vi "Modbus Property Names.vi"() -> ()   [LabVIEW 2013, in "Modbus Shared.lvlib"]
uses:
  Shared/Modbus Shared.lvlib
panel:
  in  "Modbus Items FIFO Indexes":string="Modbus Items FIFO Indexes"
  in  "Modbus Items Channels References":string="Modbus Items Channels References"
  in  "Modbus Items":string="Modbus Items"
  in  "Modbus General Settings":string="Modbus General Settings"
  in  "Modbus Configuration File Content":string="Modbus Configuration File Content"
  in  "Modbus Configuration File Path":string="Modbus Configuration File Path"
  in  "Modbus Configuration File MD5":string="Modbus Configuration File MD5"
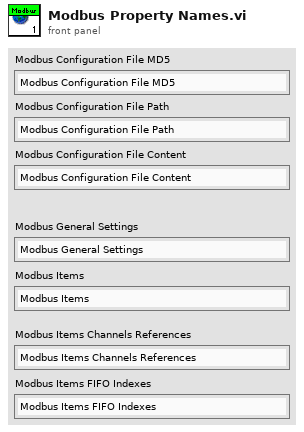
[diagram p1: front panel]
diagram:
